vi "Stop.vi"(8 "error in (no error)":errorcluster, 11 "EventDaemon in":refnum<class "ErrorHandler.lvclass">) -> (0 "error out":errorcluster, 3 "EventDaemon out":refnum<class "ErrorHandler.lvclass">)   [LabVIEW 2024, in "ErrorHandler.lvclass"]
doc: "Sends stop event to daemon."
uses:
  ErrorHandler.lvclass
  ErrorHandler.lvclass/ErrorHandler.ctl
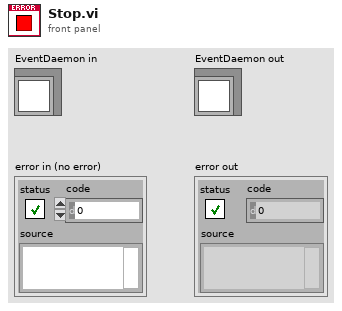
[diagram p1: front panel]
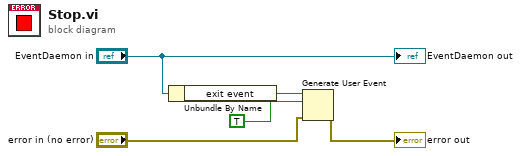
[diagram p0: block diagram]
diagram:
  n1 = Unbundle By Name("EventDaemon in") -> ("exit event"=w5:refnum<user-event>)
  n2 = Generate User Event(user event=w5, event data cluster=TRUE ("event data"), error in="error in (no error)") -> (error out=→"error out":errorcluster)  [unwired: 1 in, 1 out]
  "EventDaemon out" <- "EventDaemon in"
